vi "Command.vi"(8 "error in (no error)":errorcluster, 10 "cmd":string, 11 "PSP-405 resource in":refnum<visa-resource-name>) -> (0 "error out":errorcluster, 2 "response":string, 3 "PSP-405 resource out":refnum<visa-resource-name>)   [LabVIEW 2017, in "GW Instek PSP-405.lvlib"]
doc: "Writes the command and reads the response."
uses:
  GW Instek PSP-405.lvlib
  <vilib>/Utility/error.llb/whitespace.ctl
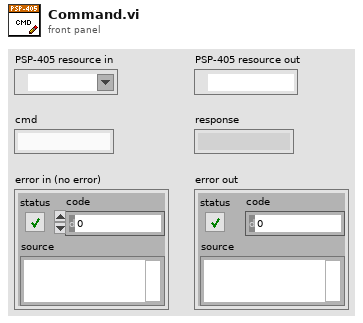
[diagram p1: front panel]
types:
  T1 = typedef "whitespace.ctl" = u16
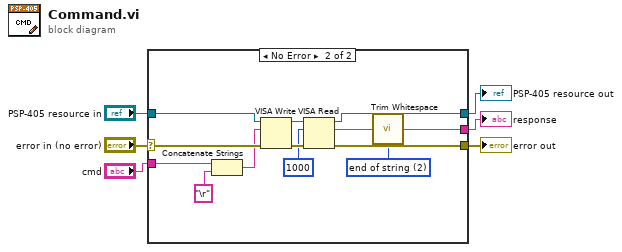
[diagram p0: block diagram]
diagram:
  n1 = case shown="No Error" "error in (no error)" {
    selector: "error in (no error)" -> [w8 w20]
    tunnel: "cmd" -> [_ w12]
    tunnel: [w8 w21] -> w4
    tunnel: [w7 w11] -> w2
    tunnel: "PSP-405 resource in" -> [w7 w10]
    tunnel: [_ w9] -> w3
    frame Error {
    }
    frame No Error {
      w15 = T1 2 items=["both", "start of string", "end of string"] ("location (both)")
      n2 = Concatenate Strings(w12, "\r" ("string")) -> (w14:string)
      n3 = VISA Write(VISA resource name=w10, write buffer=w14, error in (no error)=w20) -> (VISA resource name out=w19:refnum<visa-resource-name>, error out=w18:errorcluster)  [unwired: 1 out]
      n4 = VISA Read(VISA resource name=w19, byte count=u32 1000, error in (no error)=w18) -> (VISA resource name out=w11:refnum<visa-resource-name>, read buffer=w16:string, error out=w21:errorcluster)  [unwired: 1 out]
      n5 = call <vilib>:"Trim Whitespace.vi"("string"=w16, "location (both)"=w15) -> ("trimmed string"=w9:string)
    }
  }
  "error out" <- w4
  "PSP-405 resource out" <- w2
  "response" <- w3
